vi "Set Channel Count.vi"(9 "number of channels":i32=1, 11 "variant in":variant) -> (3 "variant out":variant)   [LabVIEW 2017]
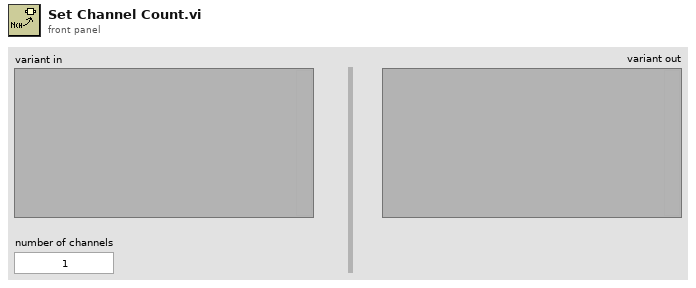
[diagram p1: front panel]
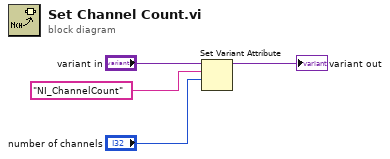
[diagram p0: block diagram]
diagram:
  n1 = Set Variant Attribute(Variant="variant in", name="NI_ChannelCount" ("TDMS property name"), value="number of channels") -> (Variant out=→"variant out":variant)  [unwired: 1 in, 2 out]
